vi "RT Main-Core_Initialize.vi"(0 "Initialization Sequence":string, 5 "FTW Actor Instance Configuration":string, 11 "error in (no error)":errorcluster) -> (4 "Actor Template-Core out":refnum<class "RT Main-Core.lvclass">, 6 "Event Refnums":T1, 15 "error out":errorcluster)   [LabVIEW 2015, in "RT Main-Core.lvclass"]
uses:
  RT Main-Core.lvclass
  source/actor/Message/Request/FTW-Message-IncomingRequest.lvclass
  source/actor/Message/Base/FTW-Message.lvclass
  RT Main-Core.lvclass/RT Main-Core.ctl
  source/CodeGen/JSON Deserialize/FTW-JSON-Deserialize.xnode
  source/CodeGen/JSON Deserialize/FTW-JSON-Core-GetFlattenedValue.vi
  source/Reflection/FTW-Reflection-Type.vi
  source/JSON/core/FTW-JSON-Core-EncodingFlags.vi
  source/JSON/FTW-JSON-Parse.vi
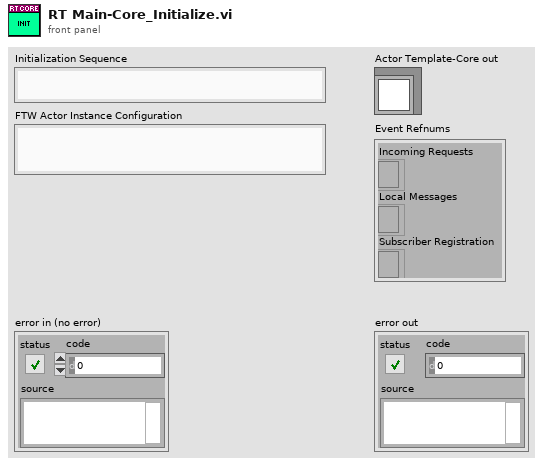
[diagram p1: front panel]
types:
  T1 = cluster{"Incoming Requests":refnum<event-registration>, "Local Messages":refnum<event-registration>, "Subscriber Registration":refnum<event-registration>}
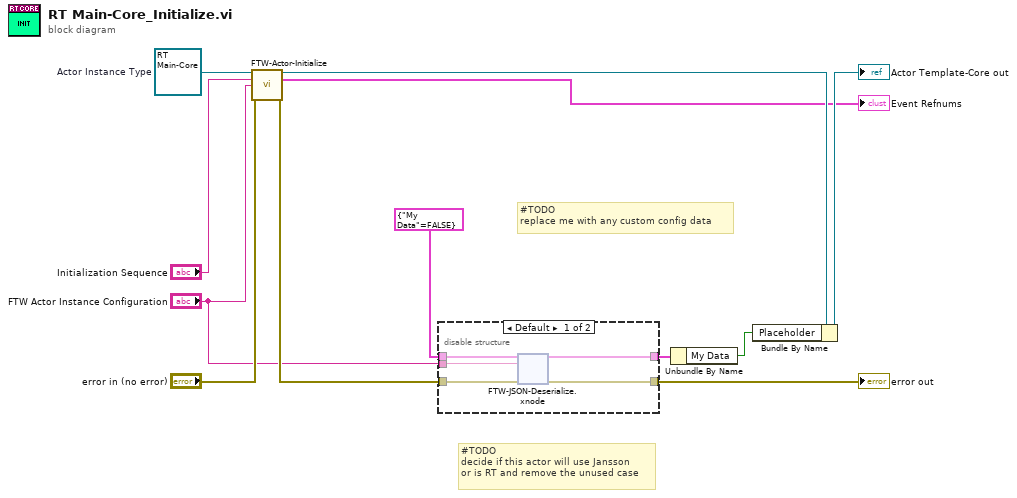
[diagram p0: block diagram]
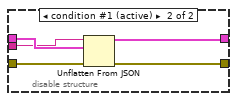
[diagram p2: hidden frame]
diagram:
  w12 = refnum<class "RT Main-Core.lvclass"> refnum  # Actor Instance Type
  # "#TODO\ndecide if this actor will use Jansson\nor is RT and remove the unused case"
  # "#TODO\nreplace me with any custom config data"
  n1 = call-dynamic "FTW-Actor-Initialize.vi"("FTW Actor Instance Type"=w12, "Initialization Job Sequence"="Initialization Sequence", "Actor Instance Configuration"="FTW Actor Instance Configuration", "error in"="error in (no error)") -> ("FTW Actor Instance"=w6:refnum<class "RT Main-Core.lvclass">, "Event Refnums"=→"Event Refnums":T1, "error out"=w4:errorcluster)  [unwired: 9 in]
  n2 = disable-structure shown="Default" {
    disable-tunnel: w4 -> [w17 w37]
    disable-tunnel: [w16 w36] -> w10
    disable-tunnel: "FTW Actor Instance Configuration" -> [w15 w34]
    disable-tunnel: cluster{"My Data":bool} {"My Data"=FALSE} ("Type and Defaults") -> [w14 w35]
    disable-tunnel: [w13 w33] -> w8
    frame condition #0 {
      n3 = xnode "FTW-JSON-Deserialize.xnode"("Type and Defaults"=w14, "JSON String"=w15, "error in"=w17) -> ("Values"=w13:cluster{"My Data":bool}, "error out"=w16:errorcluster)
    }
    frame condition #1 (active) {
      n4 = Unflatten From JSON(JSON string=w34, type and defaults=w35, error in (no error)=w37) -> (value=w33:cluster{"My Data":bool}, error out=w36:errorcluster)  [unwired: 4 in]
    }
  }
  "error out" <- w10
  n5 = Unbundle By Name(w8) -> ("My Data"=w7:bool)
  n6 = Bundle By Name(cluster=w6, "Placeholder"=w7) -> (→"Actor Template-Core out":refnum<class "RT Main-Core.lvclass">)
